vi "Send SMS example 2012.vi"() -> ()   [LabVIEW 2012]
panel:
  in  "show errors":bool
  in  "sendbutton":bool
  in  "stop":bool
  in  "email username":string
  in  "password":string
  in  "smtp server":string="smtp.gmail.com"
  in  "phone number":string
  in  "Subject":string
  in  "Carrier":enum16{"T-Mobile", "AT&T", "Verizon", "Sprint"}(ring)
  in  "Body":string
  # "1. Enter username and password for the smtp server you will be using. For gmail, be sure to include @gmail.com in the username\n\n2. Enter the phone number of the recipient including area code, no spaces or dashes.\nex: 1234567890\n\n3. Select the carrier of the recipient\n\n4. Enter a subject and body"
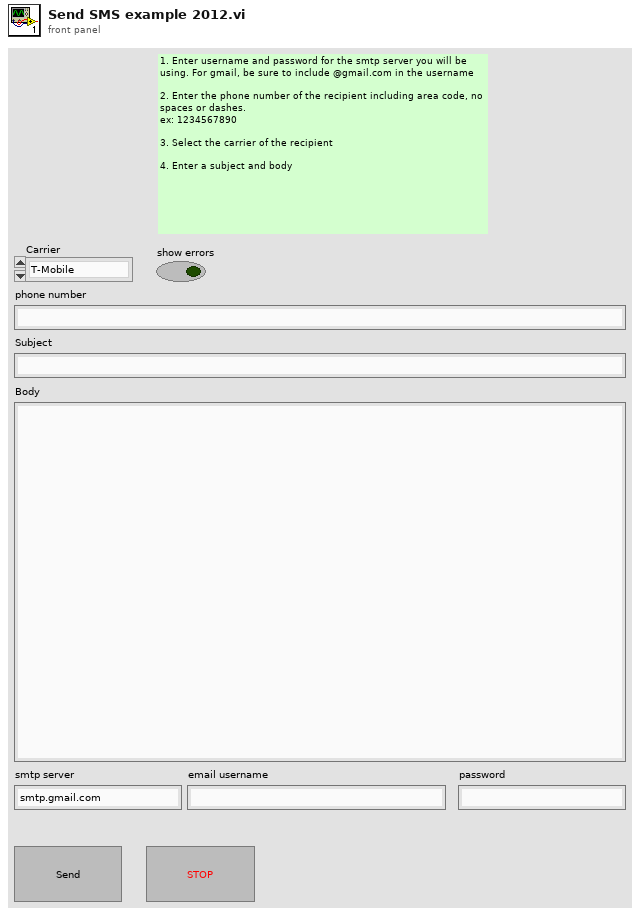
[diagram p1: front panel]
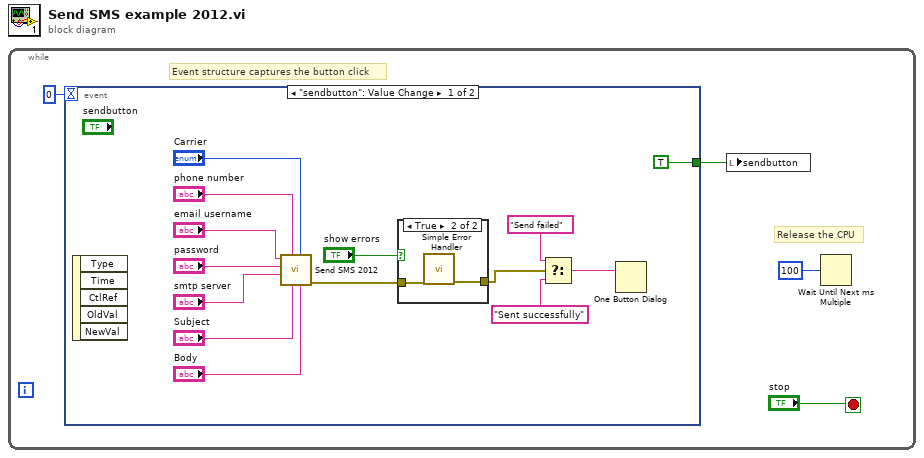
[diagram p0: block diagram]
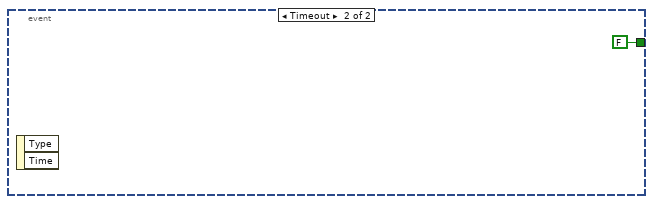
[diagram p3: hidden frame]
diagram:
  n1 = while {
    stop <- "stop" stop-if-true
    # "Release the CPU"
    # "Event structure captures the button click"
    n2 = event shown="[0] \"sendbutton\": Value Change" {
      selector: _ -> [_ _]
      dyn-events: _ -> [_ _]
      timeout: 0 -> [_ _]
      tunnel: [TRUE ("sendbutton") FALSE ("sendbutton")] -> w3
      event "sendbutton": Value Change {
        n3 = event-data() -> ()  [unwired: 1 in, 5 out]
        n4 = call "Send SMS 2012.vi"("Body"="Body", "Carrier"="Carrier", "Subject"="Subject", "phone number"="phone number", "smtp server"="smtp server", "password"="password", "email username"="email username") -> ("Error Out"=w7:errorcluster)  [unwired: 4 in]
        n5 = case shown="True" "show errors" {
          tunnel: w7 -> [w19 w21]
          tunnel: [w19 w20] -> w6
          frame False {
          }
          frame True {
            n6 = call <vilib>:"Simple Error Handler.vi"("error in (no error)"=w21) -> ("error out"=w20:errorcluster)  [unwired: 4 in, 4 out]
          }
        }
        n7 = Select(t="Send failed", s=w6, f="Sent successfully") -> (s? t:f=w9:string)
        n8 = One Button Dialog(message=w9) -> ()  [unwired: 1 in, 1 out]
      }
      event Timeout {
        n9 = event-data() -> ()  [unwired: 1 in, 2 out]
      }
    }
    n10 = local write "sendbutton"(w3) -> ()
    n11 = Wait Until Next ms Multiple(millisecond multiple=u32 100 ("milliseconds to wait")) -> ()  [unwired: 1 out]
  }
